vi "Create Data Image.vi"(8 "error in (no error)":errorcluster, 10 "Measurement":string caption="Measurement (all)", 11 "Weather Data":T2[](array[typedef])) -> (0 "error out":errorcluster, 3 "image data":T1)   [LabVIEW 2023]
doc: "HTTP method VI that retrieves all of the weather data and outputs it using stream mode. The output format is determined by the Format input terminal."
uses:
  Application/Weather Data.ctl
  <vilib>/picture/picture.llb/imagedata.ctl
  Application/Weather Data.lvlib
panel:
  out "Wind Direction":cluster{i32[], dbl[]}(graph)
  out "Wind Speed":cluster{i32[], dbl[]}(graph)
  out "Pressure":cluster{i32[], dbl[]}(graph)
  out "Temperature":cluster{i32[], dbl[]}(graph)
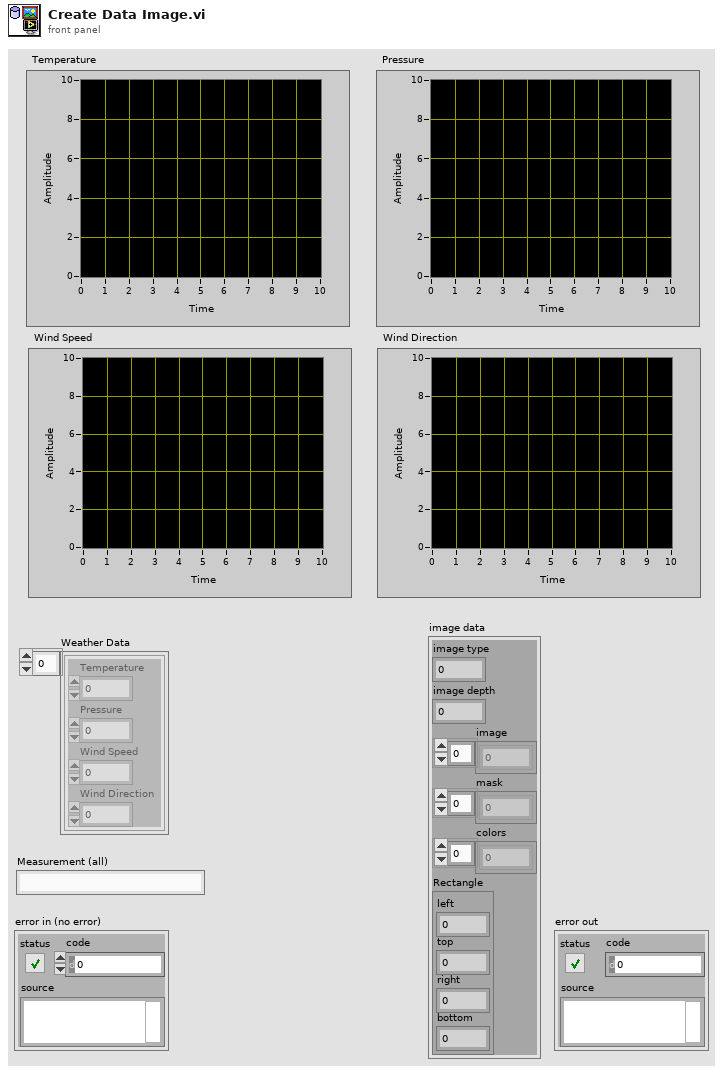
[diagram p1: front panel]
types:
  T1 = typedef "imagedata.ctl" = cluster{"image type":i32, "image depth":i32, "image":u8[], "mask":u8[], "colors":u32[], "Rectangle":cluster{"left":i16, "top":i16, "right":i16, "bottom":i16}}
  T2 = typedef "Weather Data.lvlib/Weather Data.ctl" = cluster{"Temperature":dbl, "Pressure":dbl, "Wind Speed":dbl, "Wind Direction":dbl}
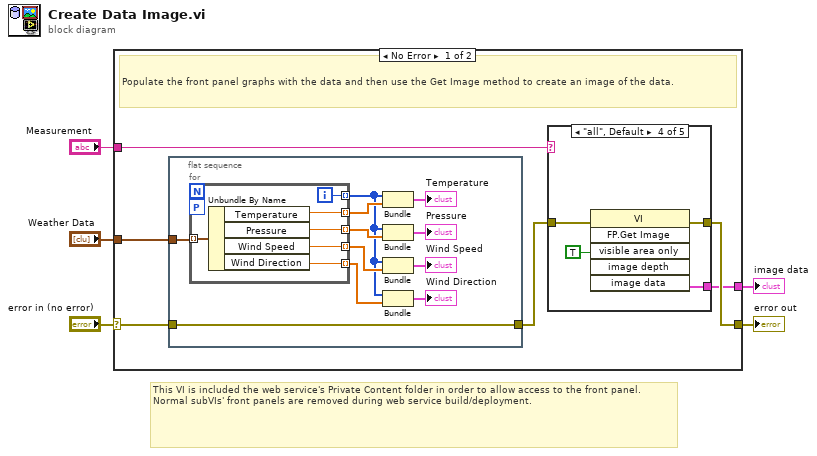
[diagram p0: block diagram]
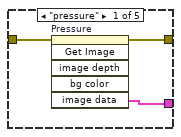
[diagram p2: hidden frame]
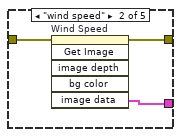
[diagram p3: hidden frame]
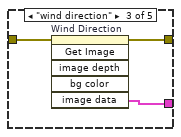
[diagram p4: hidden frame]
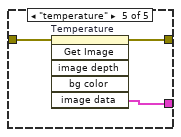
[diagram p5: hidden frame]
diagram:
  # "This VI is included the web service's Private Content folder in order to allow access to the front panel. Normal subVIs' front panels are removed during web service build/deployment."
  n1 = case shown="No Error" "error in (no error)" {
    selector: "error in (no error)" -> [w10 w45]
    tunnel: "Weather Data" -> [w11 _]
    tunnel: "Measurement" -> [w9 _]
    tunnel: [w7 w45] -> w3
    tunnel: [w6 _] -> w2
    frame No Error {
      # "Populate the front panel graphs with the data and then use the Get Image method to create an image of the data."
      n2 = flat-sequence {
        tunnel: [w21] -> w8
        tunnel: w11 -> [w22]
        tunnel: w10 -> [w21]
        frame #0 {
          n3 = for {
            tunnel: w22 -> [w28] mode=indexing
            tunnel: [w27] -> w13 mode=indexing
            tunnel: [w26] -> w20 mode=indexing
            tunnel: [w25] -> w18 mode=indexing
            tunnel: [w24] -> w15 mode=indexing
            tunnel: [w23] -> w12 mode=indexing
            workers-P: _ -> [_]
            i -> [w27]
            n4 = Unbundle By Name(w28) -> ("Temperature"=w26:dbl, "Pressure"=w25:dbl, "Wind Speed"=w24:dbl, "Wind Direction"=w23:dbl)
          }
          n5 = Bundle(w13, w20) -> (→"Temperature":cluster{i32[], dbl[]})  [unwired: 1 in]
          n6 = Bundle(w13, w18) -> (→"Pressure":cluster{i32[], dbl[]})  [unwired: 1 in]
          n7 = Bundle(w13, w15) -> (→"Wind Speed":cluster{i32[], dbl[]})  [unwired: 1 in]
          n8 = Bundle(w13, w12) -> (→"Wind Direction":cluster{i32[], dbl[]})  [unwired: 1 in]
        }
      }
      n9 = case shown="\"all\", Default" w9 {
        tunnel: w8 -> [w29 w32 w35 w39 w44]
        tunnel: [w31 w34 w37 w40 w43] -> w7
        tunnel: [w30 w33 w36 w41 w42] -> w6
        frame "pressure" {
          n10 = invoke on="Pressure" class="XYGraph (strict)" method="Get Image"(error in=w29) -> (error out=w31:errorcluster, "image data"=w30:T1)  [unwired: 5 in, 4 out]
        }
        frame "wind speed" {
          n11 = invoke on="Wind Speed" class="XYGraph (strict)" method="Get Image"(error in=w32) -> (error out=w34:errorcluster, "image data"=w33:T1)  [unwired: 5 in, 4 out]
        }
        frame "wind direction" {
          n12 = invoke on="Wind Direction" class="XYGraph (strict)" method="Get Image"(error in=w35) -> (error out=w37:errorcluster, "image data"=w36:T1)  [unwired: 5 in, 4 out]
        }
        frame "all", Default {
          n13 = invoke class="VI" method="FP.Get Image"(error in=w39, "visible area only"=TRUE ("Visible Area Only")) -> (error out=w40:errorcluster, "image data"=w41:T1)  [unwired: 4 in, 4 out]
        }
        frame "temperature" {
          n14 = invoke on="Temperature" class="XYGraph (strict)" method="Get Image"(error in=w44) -> (error out=w43:errorcluster, "image data"=w42:T1)  [unwired: 5 in, 4 out]
        }
      }
    }
    frame Error {
    }
  }
  "error out" <- w3
  "image data" <- w2
